vi "test-MecaDrvPoseEst2-testFollowTrajectory.vi"(0 "chassisSpeedsGenerator":refnum<vi>, 1 "TRAJECTORY":T11 {"States"."POSE"."ROTATION"."SIN" format="%13.4f"; "States"."POSE"."ROTATION"."COS" format="%13.4f"; "States"."POSE"."ROTATION"."VALUE" format="%13.4f"; "States"."POSE"."TRANSLATION"."Y" format="%14.3f"; "States"."POSE"."TRANSLATION"."X" format="%14.3f"; "TotalTImeSecs" format="%20.3f"}, 2 "MecaDrivePoseEstimate2":T5={"M_Vision_K"=[], "m_nominal_dT"=0.0, "m_PrevTime_Sec"=0.0, "Pose_Buffer"={"TimeStamps"=[], "DataArray"=[], "Min_TimeStamp"=0.0, "Max_TimeStamp"=0.0, "ItemCount"=0, "MaxBufferTime"=0.0}, "Meca_Drive_Odom"={"POSE"={"TRANSLATION"={"X"=0.0, "Y"=0.0}, "ROTATION"={"VALUE"=0.0, "COS"=1.0, "SIN"=0.0}}, "GyroOffset"={"VALUE"=0.0, "COS"=1.0, "SIN"=0.0}, "PreviousAngle"={"VALUE"=0.0, "COS"=1.0, "SIN"=0.0}, "Kinematics"={"FrontLeft"={"X"=0.0, "Y"=0.0}, "FrontRight"={"X"=0.0, "Y"=0.0}, "RearLeft"={"X"=0.0, "Y"=0.0}, "RearRight"={"X"=0.0, "Y"=0.0}, "InverseKinematics"=[[0.0, 1.0, -1.0, 0.0], [0.0, 1.0, 1.0, 0.0], [0.0, 1.0, 1.0, 0.0], [0.0, 1.0, -1.0, 0.0]], "ForwardKinematics"=[[0.0, 1.0, -1.0, 0.0], [0.0, 1.0, 1.0, 0.0], [0.0, 1.0, 1.0, 0.0], [0.0, 1.0, -1.0, 0.0]], "PrevCoR"={"X"=0.0, "Y"=0.0}}, "PreviousWheelPositions"={"FrontLeft"=0.0, "FrontRight"=0.0, "RearLeft"=0.0, "RearRight"=0.0, "P"=FALSE}}, "M_Q"=[[0.0], [0.0], [0.0]]} {"Meca_Drive_Odom"."PreviousWheelPositions"."RearRight" format="%19.3f"; "Meca_Drive_Odom"."PreviousWheelPositions"."RearLeft" format="%19.3f"; "Meca_Drive_Odom"."PreviousWheelPositions"."FrontRight" format="%19.3f"; "Meca_Drive_Odom"."PreviousWheelPositions"."FrontLeft" format="%19.3f"; "Meca_Drive_Odom"."Kinematics"."PrevCoR"."Y" format="%14.3f"; "Meca_Drive_Odom"."Kinematics"."PrevCoR"."X" format="%14.3f"; "Meca_Drive_Odom"."Kinematics"."RearRight"."Y" format="%14.3f"; "Meca_Drive_Odom"."Kinematics"."RearRight"."X" format="%14.3f"; "Meca_Drive_Odom"."Kinematics"."RearLeft"."Y" format="%14.3f"; "Meca_Drive_Odom"."Kinematics"."RearLeft"."X" format="%14.3f"; "Meca_Drive_Odom"."Kinematics"."FrontRight"."Y" format="%14.3f"; "Meca_Drive_Odom"."Kinematics"."FrontRight"."X" format="%14.3f"; "Meca_Drive_Odom"."Kinematics"."FrontLeft"."Y" format="%14.3f"; "Meca_Drive_Odom"."Kinematics"."FrontLeft"."X" format="%14.3f"; "Meca_Drive_Odom"."PreviousAngle"."SIN" format="%13.4f"; "Meca_Drive_Odom"."PreviousAngle"."COS" format="%13.4f"; "Meca_Drive_Odom"."PreviousAngle"."VALUE" format="%13.4f"; "Meca_Drive_Odom"."GyroOffset"."SIN" format="%13.4f"; "Meca_Drive_Odom"."GyroOffset"."COS" format="%13.4f"; "Meca_Drive_Odom"."GyroOffset"."VALUE" format="%13.4f"; "Meca_Drive_Odom"."POSE"."ROTATION"."SIN" format="%13.4f"; "Meca_Drive_Odom"."POSE"."ROTATION"."COS" format="%13.4f"; "Meca_Drive_Odom"."POSE"."ROTATION"."VALUE" format="%13.4f"; "Meca_Drive_Odom"."POSE"."TRANSLATION"."Y" format="%14.3f"; "Meca_Drive_Odom"."POSE"."TRANSLATION"."X" format="%14.3f"}, 5 "genVisionMeasurement":refnum<vi>, 7 "StartingPose":T2={"TRANSLATION"={"X"=0.0, "Y"=0.0}, "ROTATION"={"VALUE"=0.0, "COS"=1.0, "SIN"=0.0}} {"ROTATION"."SIN" format="%13.4f"; "ROTATION"."COS" format="%13.4f"; "ROTATION"."VALUE" format="%13.4f"; "TRANSLATION"."Y" format="%14.3f"; "TRANSLATION"."X" format="%14.3f"}, 9 "EndingPose":T2={"TRANSLATION"={"X"=0.0, "Y"=0.0}, "ROTATION"={"VALUE"=0.0, "COS"=1.0, "SIN"=0.0}} {"ROTATION"."SIN" format="%13.4f"; "ROTATION"."COS" format="%13.4f"; "ROTATION"."VALUE" format="%13.4f"; "TRANSLATION"."Y" format="%14.3f"; "TRANSLATION"."X" format="%14.3f"}, 11 "dt_Seconds":dbl, 12 "VisionUpdateRate":dbl, 13 "VisionUpdateDelay":dbl, 14 "CheckError":bool) -> (4 "Test Passed":bool, 6 "Output Data":T1, 15 "DataForGraph":cluster{dbl[], dbl[]}[](array[cluster]))   [LabVIEW 2019]
uses:
  <vilib>/Rock Robotics/WPI/ThirdParty/JAS_Junk/TrajLib/TypeDef/TRAJECTORY.ctl
  <vilib>/Rock Robotics/WPI/ThirdParty/JAS_Junk/TrajLib/TypeDef/TRAJ_STATE.ctl
  <vilib>/Rock Robotics/WPI/ThirdParty/JAS_Junk/TrajLib/TypeDef/POSE2D.ctl
  <vilib>/Rock Robotics/WPI/ThirdParty/JAS_Junk/TrajLib/TypeDef/TRANSLATION2D.ctl
  <vilib>/Rock Robotics/WPI/ThirdParty/JAS_Junk/TrajLib/TypeDef/ROTATION2D.ctl
  <vilib>/Rock Robotics/WPI/ThirdParty/JAS_Junk/TrajLib/TypeDef/MECA_DRIVE_POSE_EST2.ctl
  <vilib>/Analysis/Matrix/Datatypes/RealMatrix.ctl
  <vilib>/Rock Robotics/WPI/ThirdParty/JAS_Junk/TrajLib/TypeDef/TIME_INTERPOLATABLE_VARIANT.ctl
  <vilib>/Rock Robotics/WPI/ThirdParty/JAS_Junk/TrajLib/TypeDef/MECA_DRIVE_ODOMETRY.ctl
  <vilib>/Rock Robotics/WPI/ThirdParty/JAS_Junk/TrajLib/TypeDef/MECA_DRIVE_KINEMATICS.ctl
  <vilib>/Rock Robotics/WPI/ThirdParty/JAS_Junk/TrajLib/TypeDef/MECA_WHEEL_POSITIONS.ctl
  <vilib>/Rock Robotics/WPI/ThirdParty/JAS_Junk/TrajLib/Conv_Deg_Radians.vi
  <vilib>/Rock Robotics/WPI/ThirdParty/JAS_Junk/TrajLib/VI/Util_GetTime_U32.vi
  <vilib>/Rock Robotics/WPI/ThirdParty/JAS_Junk/TrajLib/Pose2d_TransformBy.vi
  <vilib>/Rock Robotics/WPI/ThirdParty/JAS_Junk/TrajLib/VI/TimeInterpPose2d_CleanUp.vi
  <vilib>/Rock Robotics/WPI/ThirdParty/JAS_Junk/TrajLib/Rotation2d_RotateBy.vi
  <vilib>/Rock Robotics/WPI/ThirdParty/JAS_Junk/TrajLib/Rotation2d_UnaryMinus.vi
  <vilib>/Rock Robotics/WPI/ThirdParty/JAS_Junk/TrajLib/Util_CalcDist.vi
  <vilib>/Rock Robotics/WPI/ThirdParty/JAS_Junk/TrajLib/Translation2d_RotateBy.vi
  <vilib>/Rock Robotics/WPI/ThirdParty/JAS_Junk/TrajLib/Translation2d_Plus.vi
  <vilib>/Rock Robotics/WPI/ThirdParty/JAS_Junk/TrajLib/Pose2d_New_TRRO.vi
  <vilib>/Rock Robotics/WPI/ThirdParty/JAS_Junk/TrajLib/Rotation2d_CreateXY.vi
  <vilib>/Rock Robotics/WPI/ThirdParty/JAS_Junk/TrajLib/VI/Util_GetTime_U64.vi
  <vilib>/gmath/interp.llb/Search Ordered Table.vi
  <vilib>/Rock Robotics/WPI/ThirdParty/JAS_Junk/TrajLib/Trajectory_Library.lvlib
  <vilib>/Analysis/Matrix/NI_Matrix.lvlib
panel:
  in  "UseVIsion":bool=TRUE
  out "error out":errorcluster
  in  "error in (no error)":errorcluster
  # "<3, 1>"
  # "<3, 3>"
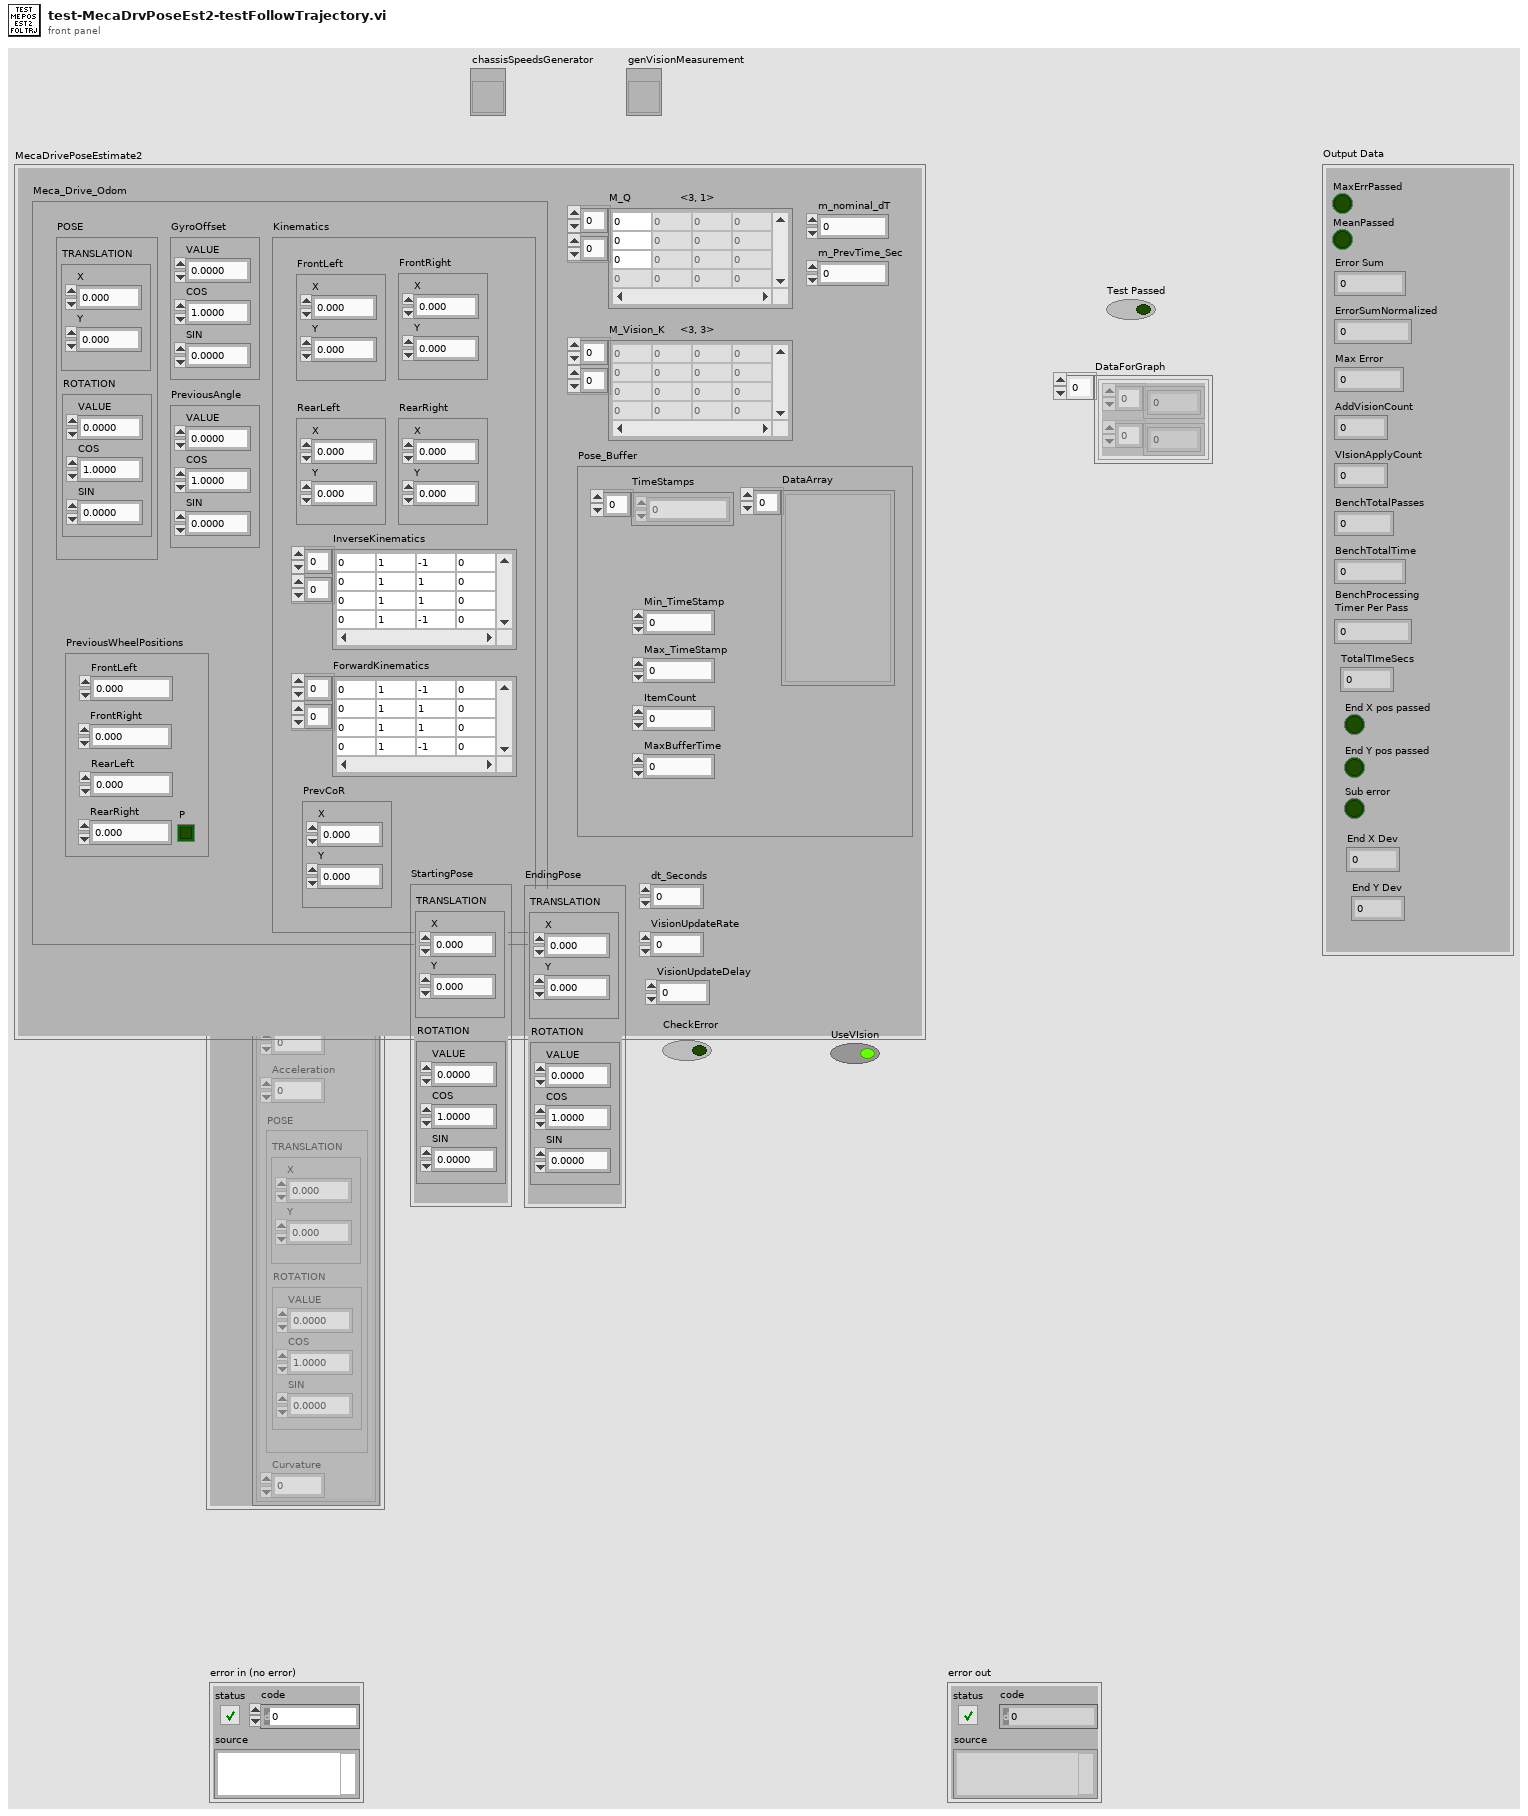
[diagram p1: front panel]
types:
  T1 = cluster{"MaxErrPassed":bool, "MeanPassed":bool, "Error Sum":dbl, "ErrorSumNormalized":dbl, "Max Error":dbl, "AddVisionCount":i32, "VIsionApplyCount":i32, "BenchTotalPasses":dbl, "BenchTotalTime":dbl, "BenchProcessing \nTimer Per Pass":dbl, "TotalTImeSecs":dbl, "End X pos passed":bool, "End Y pos passed":bool, "Sub error":bool, "End X Dev":dbl, "End Y Dev":dbl}
  T2 = typedef "Trajectory_Library.lvlib/POSE2D.ctl" = cluster{"TRANSLATION":T3, "ROTATION":T4}
  T3 = typedef "Trajectory_Library.lvlib/TRANSLATION2D.ctl" = cluster{"X":dbl, "Y":dbl}
  T4 = typedef "Trajectory_Library.lvlib/ROTATION2D.ctl" = cluster{"VALUE":dbl, "COS":dbl, "SIN":dbl}
  T5 = typedef "Trajectory_Library.lvlib/MECA_DRIVE_POSE_EST2.ctl" = cluster{"M_Vision_K":T6, "m_nominal_dT":dbl, "m_PrevTime_Sec":dbl, "Pose_Buffer":T7, "Meca_Drive_Odom":T8, "M_Q":T6}
  T6 = typedef "NI_Matrix.lvlib/RealMatrix.ctl" = dbl[][]
  T7 = typedef "Trajectory_Library.lvlib/TIME_INTERPOLATABLE_VARIANT.ctl" = cluster{"TimeStamps":dbl[], "DataArray":variant[], "Min_TimeStamp":dbl, "Max_TimeStamp":dbl, "ItemCount":i32, "MaxBufferTime":dbl}
  T8 = typedef "Trajectory_Library.lvlib/MECA_DRIVE_ODOMETRY.ctl" = cluster{"POSE":T2, "GyroOffset":T4, "PreviousAngle":T4, "Kinematics":T9, "PreviousWheelPositions":T10}
  T9 = typedef "Trajectory_Library.lvlib/MECA_DRIVE_KINEMATICS.ctl" = cluster{"FrontLeft":T3, "FrontRight":T3, "RearLeft":T3, "RearRight":T3, "InverseKinematics":T6, "ForwardKinematics":T6, "PrevCoR":T3}
  T10 = typedef "Trajectory_Library.lvlib/MECA_WHEEL_POSITIONS.ctl" = cluster{"FrontLeft":dbl, "FrontRight":dbl, "RearLeft":dbl, "RearRight":dbl, "P":bool}
  T11 = typedef "Trajectory_Library.lvlib/TRAJECTORY.ctl" = cluster{"TotalTImeSecs":dbl, "States":T12[]}
  T12 = typedef "Trajectory_Library.lvlib/TRAJ_STATE.ctl" = cluster{"TimeSeconds":dbl, "Velocity":dbl, "Acceleration":dbl, "POSE":T2, "Curvature":dbl}
  T13 = typedef "Trajectory_Library.lvlib/TIME_INTERPOLATABLE_POSE2D.ctl" = cluster{"TimeStamps":dbl[], "Pose":T2[], "Min_TimeStamp":dbl, "Max_TimeStamp":dbl, "ItemCount":i32, "MaxBufferTime":dbl}
  T14 = typedef "Trajectory_Library.lvlib/TRANSFORM2D.ctl" = cluster{"TRANSLATION":T3, "ROTATION":T4, "xF":bool}
  T15 = typedef "Trajectory_Library.lvlib/CHASSIS_SPEEDS.ctl" = cluster{"vX":dbl, "vY":dbl, "vOmega":dbl}
  T16 = typedef "Trajectory_Library.lvlib/MECA_WHEEL_SPEEDS.ctl" = cluster{"FrontLeftSpeed":dbl, "FrontRightSpeed":dbl, "RearLeftSpeed":dbl, "RearRightSpeed":dbl}
  T17 = cluster{bool, bool, "Error Sum":dbl, dbl, dbl, i32, i32, "TotalPasses":dbl, "TotalTime":dbl, dbl, "TotalTImeSecs":dbl, bool, bool, bool, dbl, dbl}
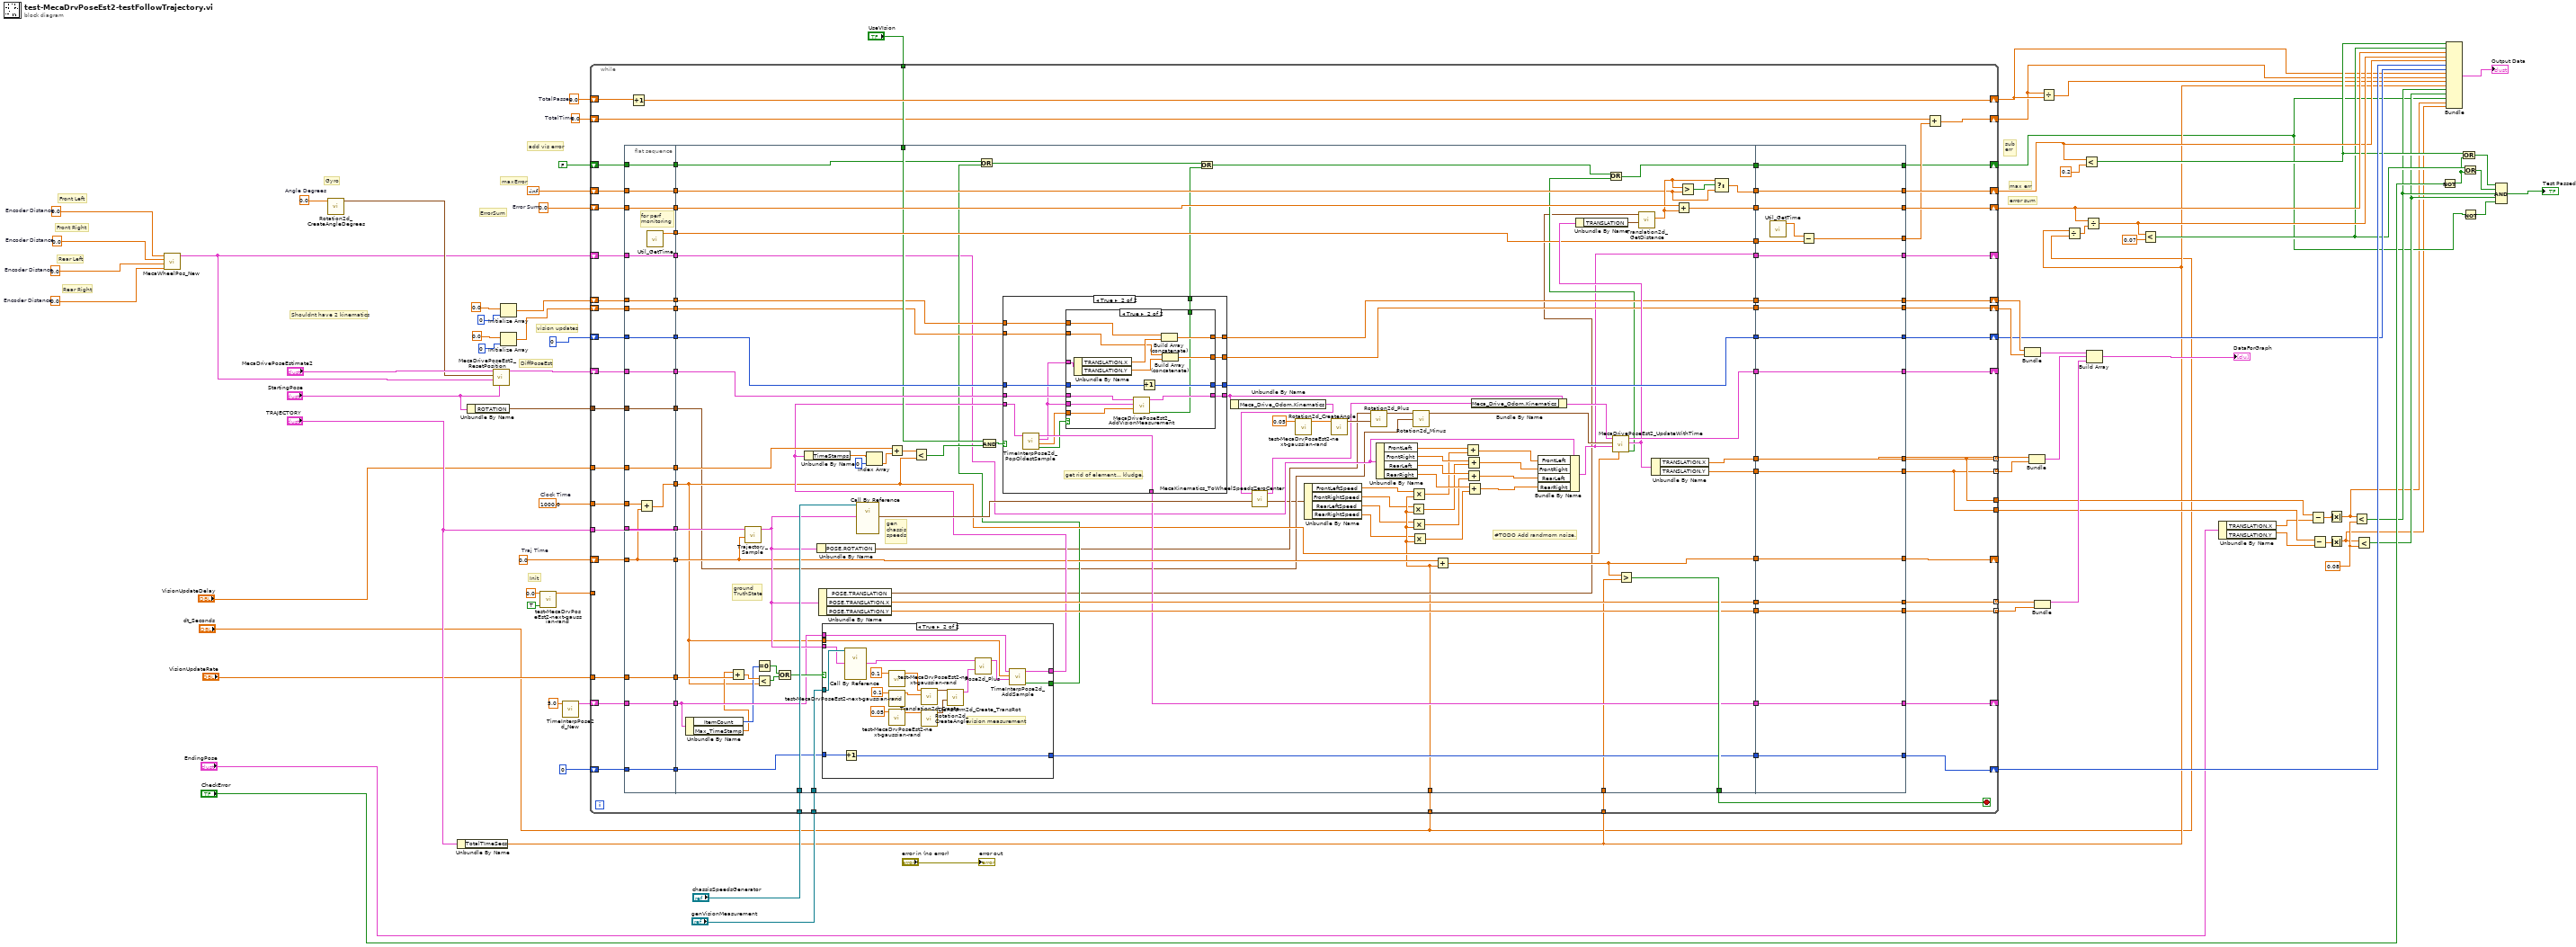
[diagram p0: block diagram]
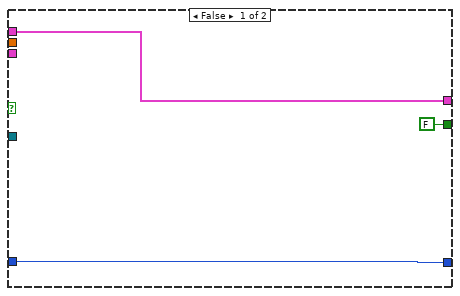
[diagram p2: hidden frame]
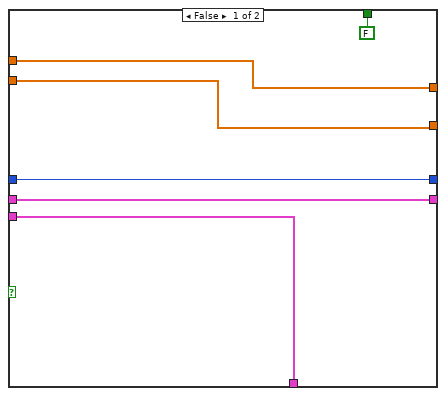
[diagram p3: hidden frame]
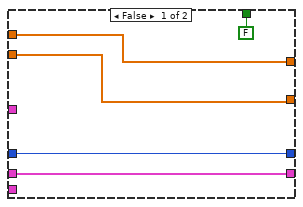
[diagram p4: hidden frame]
diagram:
  w1 = 0.0  # Encoder Distance
  w2 = 0.0  # Encoder Distance
  w3 = 0.0  # Encoder Distance
  w4 = 0.0  # Encoder Distance
  w27 = 0.08
  w52 = 1000.0  # Clock Time
  w60 = 0.0  # Angle Degrees
  w80 = 0.0  # TotalPasses
  w79 = 0.0  # TotalTime
  w74 = 0.0  # Error Sum
  w64 = 0.0  # Traj Time
  # "Shouldnt have 2 kinematics"
  # "Front Left"
  # "Rear Right"
  # "Rear Left"
  # "Front Right"
  # "Init"
  # "sub\nerr"
  # "add vis error"
  # "max err"
  # "error sum"
  # "Gyro"
  # "ErrorSum"
  # "maxError"
  # "vision updates"
  # "DiffPoseEst"
  n1 = call <vilib>:"MecaWheelPos_New.vi"("RearRightPosition"=w1, "RearLeftPosition"=w2, "FrontRightPosition"=w3, "FrontLeftPosition"=w4) -> ("MECA_WHEEL_POSITIONS"=w5:T10)  [unwired: 7 in]
  n2 = call <vilib>:"Rotation2d_CreateAngleDegrees.vi"("Angle_Degrees"=w60) -> ("ROTATION"=w59:T4)  [unwired: 10 in]
  n3 = Unbundle By Name("TRAJECTORY") -> ("TotalTImeSecs"=w17:dbl)
  n4 = Unbundle By Name("StartingPose") -> ("ROTATION"=w35:T4)
  n5 = call <vilib>:"MecaDrivePoseEst2_ResetPosition.vi"("Pose"="StartingPose", "Module Positions"=w5, "Gyro"=w59, "in MecaDrivePoseEst2"="MecaDrivePoseEstimate2") -> ("Out MecaDrivePoseEst2"=w61:T5)  [unwired: 7 in]
  n6 = Initialize Array(0.0, 0 ("dimension size")) -> (w47:dbl[])
  n7 = Initialize Array(0.0, 0 ("dimension size")) -> (w46:dbl[])
  n8 = call "test-MecaDrvPoseEst2-next-gaussian-rand.vi"("Init"=TRUE, "Multiplier"=0.0 ("R2")) -> ("Gaussian white noise"=w6:dbl)  [unwired: 9 in]
  n9 = call <vilib>:"TimeInterpPose2d_New.vi"("MaxTime"=5.0) -> ("TimeInterpPose"=w56:T13)  [unwired: 10 in]
  n10 = while {
    shift-right: [w158] -> _
    shift-left: w64 -> [w154]
    tunnel: "TRAJECTORY" -> [w156]
    tunnel: w17 -> [w157]
    tunnel: "VisionUpdateRate" -> [w112]
    shift-right: [w123] -> _
    shift-left: w61 -> [w155]
    tunnel: [w94] -> w65 mode=indexing
    tunnel: [w93] -> w66 mode=indexing
    shift-right: [w152] -> w37
    shift-left: 0 -> [w153]
    tunnel: [w151] -> w70 mode=indexing
    tunnel: [w150] -> w71 mode=indexing
    shift-right: [w147] -> w40
    shift-left: -inf -> [w146]
    shift-right: [w148] -> w42
    shift-left: w74 -> [w149]
    shift-right: [w89] -> w19
    shift-left: w79 -> [w90]
    shift-right: [w125] -> w20
    shift-left: w80 -> [w126]
    tunnel: "UseVIsion" -> [w124]
    shift-right: [w120] -> _
    shift-left: w5 -> [w121]
    shift-right: [w115] -> _
    shift-left: w56 -> [w117]
    tunnel: "chassisSpeedsGenerator" -> [w118]
    tunnel: "genVisionMeasurement" -> [w113]
    tunnel: "VisionUpdateDelay" -> [w111]
    tunnel: w52 -> [w109]
    shift-right: [w104] -> w45
    shift-left: w47 -> [w107]
    shift-right: [w102] -> w44
    shift-left: w46 -> [w105]
    shift-right: [w98] -> w38
    shift-left: 0 -> [w99]
    tunnel: w35 -> [w95]
    tunnel: [w94] -> w33
    tunnel: [w93] -> w32
    shift-right: [w86] -> w12
    shift-left: FALSE -> [w87]
    tunnel: "dt_Seconds" -> [w84]
    tunnel: w6 -> [_]
    stop <- w145 stop-if-true
    n11 = flat-sequence {
      tunnel: w146 -> [w171]
      tunnel: w149 -> [w172]
      tunnel: w153 -> [w173]
      tunnel: w154 -> [w165]
      tunnel: w155 -> [w174]
      tunnel: w112 -> [w175]
      tunnel: w156 -> [w176]
      tunnel: [w176] -> w144
      tunnel: [w175] -> w143
      tunnel: [w174] -> w142
      tunnel: [w165] -> w141
      tunnel: [w173] -> w140
      tunnel: [w172] -> w139
      tunnel: [w171] -> w138
      tunnel: [w167] -> w128
      tunnel: [w170] -> w122
      tunnel: w121 -> [w170]
      tunnel: w117 -> [w169]
      tunnel: [w169] -> w116
      tunnel: w111 -> [w168]
      tunnel: [w168] -> w110
      tunnel: w109 -> [w166]
      tunnel: [w164] -> w108
      tunnel: w107 -> [w164]
      tunnel: [w163] -> w106
      tunnel: w105 -> [w163]
      tunnel: [w162] -> w100
      tunnel: w99 -> [w162]
      tunnel: [w161] -> w96
      tunnel: w95 -> [w161]
      tunnel: [w160] -> w92
      tunnel: [w159] -> w88
      tunnel: w87 -> [w159]
      tunnel: [w266] -> w145
      tunnel: w157 -> [w212]
      tunnel: w144 -> [w264]
      tunnel: w143 -> [w238]
      tunnel: w142 -> [w263]
      tunnel: w141 -> [w224]
      tunnel: w140 -> [w259]
      tunnel: w139 -> [w253]
      tunnel: w138 -> [w211]
      tunnel: [w265] -> w137
      tunnel: [w262] -> w136
      tunnel: [w261] -> w135
      tunnel: [w260] -> w134
      tunnel: [w258] -> w133
      tunnel: [w257] -> w132
      tunnel: [w256] -> w131
      tunnel: [w252] -> w130
      tunnel: [w249] -> w129
      tunnel: w128 -> [w248]
      tunnel: [w248] -> w127
      tunnel: w124 -> [w232]
      tunnel: w122 -> [w198]
      tunnel: [w199] -> w119
      tunnel: w118 -> [w245]
      tunnel: w116 -> [w236]
      tunnel: [w223] -> w114
      tunnel: w113 -> [w243]
      tunnel: w110 -> [w229]
      tunnel: w108 -> [w222]
      tunnel: w106 -> [w221]
      tunnel: [w220] -> w103
      tunnel: [w219] -> w101
      tunnel: w100 -> [w218]
      tunnel: [w217] -> w97
      tunnel: w96 -> [w194]
      tunnel: w92 -> [w213]
      tunnel: w88 -> [w206]
      tunnel: [w208] -> w85
      tunnel: w84 -> [w191]
      tunnel: [w337] -> w147
      tunnel: [w338] -> w148
      tunnel: [w339] -> w150
      tunnel: [w340] -> w151
      tunnel: [w341] -> w152
      tunnel: [w342] -> w93
      tunnel: [w343] -> w94
      tunnel: [w344] -> w123
      tunnel: [w345] -> w158
      tunnel: w137 -> [w345]
      tunnel: w136 -> [w344]
      tunnel: w135 -> [w343]
      tunnel: w134 -> [w342]
      tunnel: w133 -> [w341]
      tunnel: w132 -> [w340]
      tunnel: w131 -> [w339]
      tunnel: w130 -> [w338]
      tunnel: w129 -> [w337]
      tunnel: w127 -> [w335]
      tunnel: [w334] -> w120
      tunnel: w119 -> [w334]
      tunnel: [w333] -> w115
      tunnel: w114 -> [w333]
      tunnel: [w332] -> w104
      tunnel: w103 -> [w332]
      tunnel: [w331] -> w102
      tunnel: w101 -> [w331]
      tunnel: [w330] -> w98
      tunnel: w97 -> [w330]
      tunnel: [w329] -> w91
      tunnel: [w328] -> w86
      tunnel: w85 -> [w328]
      frame #0 {
        # "for perf\nmonitoring"
        n12 = Add(x=w166, y=w165) -> (x+y=w160:dbl)
        n13 = call <vilib>:"Util_GetTime.vi"() -> ("FPGA_Time_Seconds"=w167:dbl)  [unwired: 9 in, 2 out]
      }
      frame #1 {
        # "#TODO Add randmom noise."
        # "gen\nchassis\nspeeds"
        # "ground\nTruthState"
        n14 = Unbundle By Name(w236) -> ("ItemCount"=w235:i32, "Max_TimeStamp"=w234:dbl)
        n15 = Add(x=w234, y=w238) -> (x+y=w237:dbl)
        n16 = call <vilib>:"Trajectory_Sample.vi"("Time"=w224, "InputTRAJECTORY"=w264) -> ("OutputTRAJ_STATE"=w242:T12)  [unwired: 9 in]
        n17 = Equal To 0?(x=w235) -> (x = 0?=w241:bool)
        n18 = Less?(x=w237, y=w213) -> (x < y?=w240:bool)
        n19 = Compound Arithmetic op=OR(w241, w240) -> (w239:bool)
        n20 = Unbundle By Name(w242) -> ("POSE.ROTATION"=w195:T4)
        n21 = Unbundle By Name(w242) -> ("POSE.TRANSLATION"=w192:T3, "POSE.TRANSLATION.X"=w256:dbl, "POSE.TRANSLATION.Y"=w257:dbl)
        n22 = case shown="True" w239 {
          tunnel: w243 -> [_ w288]
          tunnel: w242 -> [_ w287]
          tunnel: w236 -> [w269 w276]
          tunnel: w213 -> [_ w274]
          tunnel: [w269 w273] -> w226
          tunnel: w218 -> [w268 w272]
          tunnel: [w268 w271] -> w217
          tunnel: [FALSE ("Error") w270] -> w204
          frame False {
          }
          frame True {
            # "vision measurement"
            n23 = Increment(x=w272) -> (x+1=w271:i32)
            n24 = call-by-ref "?"(reference=w288, "TRAJ_STATE"=w287) -> ("POSE2D"=w286:T2)  [unwired: 11 in, 2 out]
            n25 = call "test-MecaDrvPoseEst2-next-gaussian-rand.vi"("Multiplier"=0.1 ("R0")) -> ("Gaussian white noise"=w281:dbl)  [unwired: 10 in]
            n26 = call "test-MecaDrvPoseEst2-next-gaussian-rand.vi"("Multiplier"=0.1 ("R1")) -> ("Gaussian white noise"=w282:dbl)  [unwired: 10 in]
            n27 = call "test-MecaDrvPoseEst2-next-gaussian-rand.vi"("Multiplier"=0.05 ("R2")) -> ("Gaussian white noise"=w283:dbl)  [unwired: 10 in]
            n28 = call <vilib>:"Translation2d_Create.vi"("Y"=w282, "X"=w281) -> ("TRANSLATION"=w284:T3)  [unwired: 9 in]
            n29 = call <vilib>:"Rotation2d_CreateAngle.vi"("Angle"=w283) -> ("ROTATION"=w285:T4)  [unwired: 10 in]
            n30 = call <vilib>:"Transform2d_Create_TransRot.vi"("ROTATION"=w285, "TRANSLATION"=w284) -> ("TRANSFORM"=w277:T14)  [unwired: 9 in]
            n31 = call <vilib>:"Pose2d_Plus.vi"("other TRANSFORM"=w277, "in POSE"=w286) -> ("out POSE"=w275:T2)  [unwired: 9 in]
            n32 = call <vilib>:"TimeInterpPose2d_AddSample.vi"("Pose"=w275, "TimeStamp"=w274, "in TimeInterpPose"=w276) -> ("Error"=w270:bool, "out TimeInterpPose"=w273:T13)  [unwired: 7 in]
          }
        }
        n33 = Unbundle By Name(w226) -> ("TimeStamps"=w231:dbl[])
        n34 = call-by-ref "?"(reference=w245, "TRAJ_STATE"=w242) -> ("CHASSIS"=w244:T15)  [unwired: 11 in, 2 out]
        n35 = Index Array(array=w231, index=0) -> (element=w225:dbl)
        n36 = Add(x=w229, y=w225) -> (x+y=w228:dbl)
        n37 = Less?(x=w228, y=w213) -> (x < y?=w227:bool)
        n38 = Or(x=w206, y=w204) -> (x .or. y?=w205:bool)
        n39 = And(x=w232, y=w227) -> (x .and. y?=w233:bool)
        n40 = case shown="True" w233 {
          tunnel: w263 -> [w294 w308]
          tunnel: [w294 w307] -> w202
          tunnel: w259 -> [w293 w303]
          tunnel: [w293 w302] -> w258
          tunnel: w226 -> [w292 w306]
          tunnel: [w292 w305] -> w223
          tunnel: w222 -> [w291 w299]
          tunnel: w221 -> [w290 w298]
          tunnel: [w291 w297] -> w220
          tunnel: [w290 w296] -> w219
          tunnel: [FALSE ("Error") w295] -> w210
          frame False {
          }
          frame True {
            # "get rid of element... kludge."
            n41 = call <vilib>:"TimeInterpPose2d_PopOldestSample.vi"("in TimeInterpPose2d"=w306) -> ("Is Present"=w304:bool, "TimeStamp"=w301:dbl, "OutputPose2d"=w300:T2, "out TimeInterpPose2d"=w305:T13)  [unwired: 7 in]
            n42 = case shown="True" w304 {
              tunnel: w308 -> [w313 w327]
              tunnel: [w313 w326] -> w307
              tunnel: w303 -> [w312 w325]
              tunnel: [w312 w324] -> w302
              tunnel: w300 -> [_ w323]
              tunnel: w301 -> [_ w322]
              tunnel: w300 -> [_ w321]
              tunnel: w299 -> [w311 w318]
              tunnel: w298 -> [w310 w317]
              tunnel: [w311 w316] -> w297
              tunnel: [w310 w315] -> w296
              tunnel: [FALSE ("Error") w314] -> w295
              frame False {
              }
              frame True {
                n43 = Unbundle By Name(w321) -> ("TRANSLATION.X"=w320:dbl, "TRANSLATION.Y"=w319:dbl)
                n44 = call <vilib>:"MecaDrivePoseEst2_AddVisionMeasurement.vi"("TImeStamp_Seconds"=w322, "visionRobotPose"=w323, "in MecaDrivePoseEst2"=w327) -> ("Error"=w314:bool, "Out MecaDrivePoseEst2"=w326:T5)  [unwired: 7 in]
                n45 = Increment(x=w325) -> (x+1=w324:i32)
                n46 = Build Array (concatenate)(w318, w320) -> (w316:dbl[])
                n47 = Build Array (concatenate)(w317, w319) -> (w315:dbl[])
              }
            }
          }
        }
        n48 = Or(x=w205, y=w210) -> (x .or. y?=w209:bool)
        n49 = Unbundle By Name(w202) -> ("Meca_Drive_Odom.Kinematics"=w203:T9)
        n50 = call <vilib>:"MecaKinematics_ToWheelSpeedsZeroCenter.vi"("ChassisSpeeds"=w244, "in MECA_DRIVE_KINEMATICS"=w203) -> ("MECA_WHEEL_SPEEDS"=w193:T16, "out MECA_DRIVE_KINEMATICS"=w200:T9)  [unwired: 8 in]
        n51 = call "test-MecaDrvPoseEst2-next-gaussian-rand.vi"("Multiplier"=0.05 ("R0")) -> ("Gaussian white noise"=w246:dbl)  [unwired: 10 in]
        n52 = Unbundle By Name(w193) -> ("FrontLeftSpeed"=w190:dbl, "FrontRightSpeed"=w189:dbl, "RearLeftSpeed"=w188:dbl, "RearRightSpeed"=w187:dbl)
        n53 = call <vilib>:"Rotation2d_CreateAngle.vi"("Angle"=w246) -> ("ROTATION"=w247:T4)  [unwired: 10 in]
        n54 = call <vilib>:"Rotation2d_Plus.vi"("other ROTATION"=w247, "in ROTATION"=w195) -> ("out ROTATION"=w216:T4)  [unwired: 9 in]
        n55 = Unbundle By Name(w198) -> ("FrontLeft"=w197:dbl, "FrontRight"=w186:dbl, "RearLeft"=w185:dbl, "RearRight"=w184:dbl)
        n56 = Multiply(x=w189, y=w191) -> (x*y=w182:dbl)
        n57 = Multiply(x=w190, y=w191) -> (x*y=w183:dbl)
        n58 = Multiply(x=w188, y=w191) -> (x*y=w181:dbl)
        n59 = Multiply(x=w187, y=w191) -> (x*y=w180:dbl)
        n60 = call <vilib>:"Rotation2d_Minus.vi"("other ROTATION"=w194, "in ROTATION"=w216) -> ("out ROTATION"=w215:T4)  [unwired: 9 in]
        n61 = Add(x=w224, y=w191) -> (x+y=w265:dbl)
        n62 = Add(x=w197, y=w183) -> (x+y=w196:dbl)
        n63 = Add(x=w186, y=w182) -> (x+y=w179:dbl)
        n64 = Add(x=w185, y=w181) -> (x+y=w178:dbl)
        n65 = Add(x=w184, y=w180) -> (x+y=w177:dbl)
        n66 = Bundle By Name(cluster=w202, "Meca_Drive_Odom.Kinematics"=w200) -> (w201:T5)
        n67 = Bundle By Name(cluster=w198, "FrontLeft"=w196, "FrontRight"=w179, "RearLeft"=w178, "RearRight"=w177) -> (w199:T10)
        n68 = call <vilib>:"MecaDrivePoseEst2_UpdateWithTime.vi"("CurrentTimeSeconds"=w213, "module Positions"=w199, "GyroAngle"=w215, "in MecaDrivePoseEst2"=w201) -> ("Error"=w207:bool, "Estimated Pose"=w255:T2, "Out MecaDrivePoseEst2"=w262:T5)  [unwired: 5 in]
        n69 = Unbundle By Name(w255) -> ("TRANSLATION"=w254:T3)
        n70 = Or(x=w209, y=w207) -> (x .or. y?=w208:bool)
        n71 = Greater?(x=w265, y=w212) -> (0:w266:bool)
        n72 = call <vilib>:"Translation2d_GetDistance.vi"("other Translation"=w254, "In Translation"=w192) -> ("Distance"=w250:dbl)  [unwired: 9 in]
        n73 = Unbundle By Name(w255) -> ("TRANSLATION.X"=w261:dbl, "TRANSLATION.Y"=w260:dbl)
        n74 = Add(x=w253, y=w250) -> (x+y=w252:dbl)
        n75 = Greater?(x=w250, y=w211) -> (0:w251:bool)
        n76 = Select(t=w250, s=w251, f=w211) -> (s? t:f=w249:dbl)
      }
      frame #2 {
        n77 = call <vilib>:"Util_GetTime.vi"() -> ("FPGA_Time_Seconds"=w336:dbl)  [unwired: 9 in, 2 out]
        n78 = Subtract(x=w336, y=w335) -> (x-y=w329:dbl)
      }
    }
    n79 = Increment(x=w126) -> (x+1=w125:dbl)
    n80 = Add(x=w90, y=w91) -> (x+y=w89:dbl)
  }
  n81 = Bundle(w45, w44) -> (w67:cluster{dbl[], dbl[]})  [unwired: 1 in]
  n82 = Bundle(w65, w66) -> (w68:cluster{dbl[], dbl[]})  [unwired: 1 in]
  n83 = Bundle(w71, w70) -> (w72:cluster{dbl[], dbl[]})  [unwired: 1 in]
  n84 = Divide(x=w19, y=w20) -> (x/y=w18:dbl)
  n85 = Divide(x=w17, y="dt_Seconds") -> (x/y=w78:dbl)
  n86 = Less?(x=w40, y=0.2) -> (x < y?=w26:bool)
  n87 = Divide(x=w42, y=w78) -> (x/y=w41:dbl)
  n88 = Build Array(w67, w68, w72) -> (→"DataForGraph":cluster{dbl[], dbl[]}[])
  n89 = Less?(x=w41, y=0.07) -> (x < y?=w25:bool)
  n90 = Unbundle By Name("EndingPose") -> ("TRANSLATION.X"=w31:dbl, "TRANSLATION.Y"=w30:dbl)
  n91 = Subtract(x=w33, y=w31) -> (x-y=w29:dbl)
  n92 = Subtract(x=w32, y=w30) -> (x-y=w28:dbl)
  n93 = Absolute Value(x=w29) -> (abs(x)=w10:dbl)
  n94 = Absolute Value(x=w28) -> (abs(x)=w9:dbl)
  n95 = Less?(x=w10, y=w27) -> (x < y?=w16:bool)
  n96 = Less?(x=w9, y=w27) -> (x < y?=w15:bool)
  n97 = Not(x="CheckError") -> (.not. x?=w24:bool)
  n98 = Bundle(w26, w25, "Error Sum"=w42, w41, w40, w38, w37, "TotalPasses"=w20, "TotalTime"=w19, w18, "TotalTImeSecs"=w17, w16, w15, w12, w10, w9) -> (→"Output Data":T17)  [unwired: 1 in]
  n99 = Or(x=w26, y=w24) -> (x .or. y?=w22:bool)
  n100 = Or(x=w25, y=w24) -> (x .or. y?=w23:bool)
  n101 = Not(x=w12) -> (.not. x?=w13:bool)
  n102 = Compound Arithmetic op=AND(w22, w23, w16, w15, w13) -> (→"Test Passed":bool)
  "error out" <- "error in (no error)"
